vi "Stiffness Jacobian DAO.vi"(7 "refnum in":T1, 8 "error in (no error)":errorcluster, 9 "Stiffness Jacobian In":T4=[[1000000.0, 0.0, 0.0, 0.0, 0.0, 0.0], [0.0, 1000000.0, 0.0, 0.0, 0.0, 0.0], [0.0, 0.0, 1000000.0, 0.0, 0.0, 0.0], [0.0, 0.0, 0.0, 1000000.0, 0.0, 0.0], [0.0, 0.0, 0.0, 0.0, 1000000.0, 0.0], [0.0, 0.0, 0.0, 0.0, 0.0, 1000000.0]], 10 "LBCB Number":T2, 11 "Actions":T3) -> (0 "error out":errorcluster, 3 "Stiffness Jacobian Out":T4=[[1000000.0, 0.0, 0.0, 0.0, 0.0, 0.0], [0.0, 1000000.0, 0.0, 0.0, 0.0, 0.0], [0.0, 0.0, 1000000.0, 0.0, 0.0, 0.0], [0.0, 0.0, 0.0, 1000000.0, 0.0, 0.0], [0.0, 0.0, 0.0, 0.0, 1000000.0, 0.0], [0.0, 0.0, 0.0, 0.0, 0.0, 1000000.0]], 4 "refnum out":T1)   [LabVIEW 2009]
uses:
  MixedMode/Stiffness Matrix.ctl
  Metadata/Persistant DAO Actions.ctl
  Metadata/LBCB Number.ctl
  <vilib>/Utility/config.llb/Config Data RefNum.ctl
  <vilib>/Utility/config.llb/NI_LVConfig.lvlib
panel:
  in  "Keys":string[](array[string])=["dFx", "dFy", "dFz", "dMx", "dMy", "dMz"]
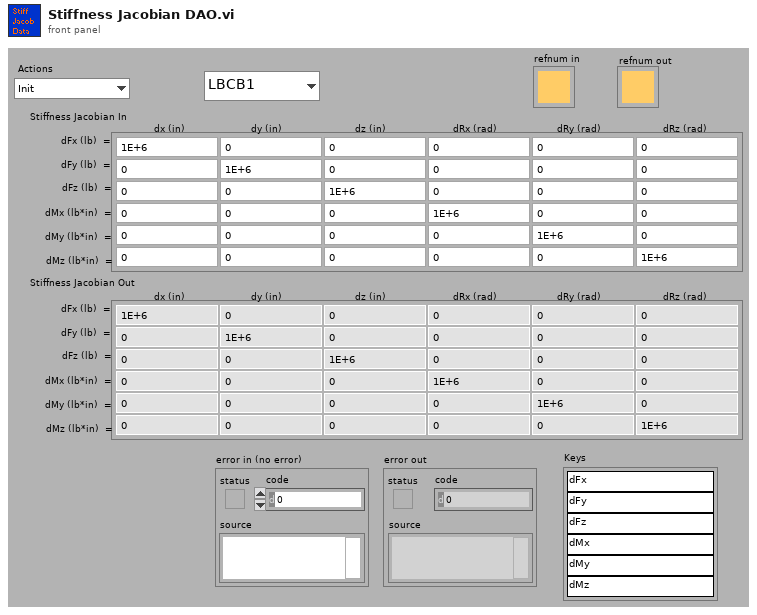
[diagram p1: front panel]
types:
  T1 = typedef "NI_LVConfig.lvlib/Config Data RefNum.ctl" = refnum<k1>
  T2 = typedef "LBCB Number.ctl" = enum16{"LBCB1", "LBCB2"}
  T3 = typedef "Persistant DAO Actions.ctl" = enum16{"Init", "Get", "Set", "Load", "Save"}
  T4 = typedef "Stiffness Matrix.ctl" = dbl[][]
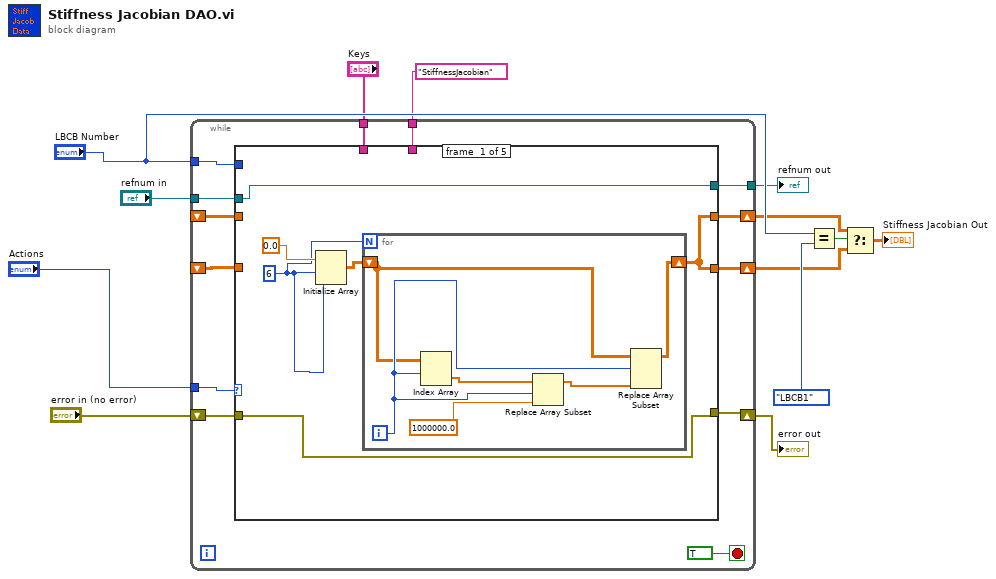
[diagram p0: block diagram]
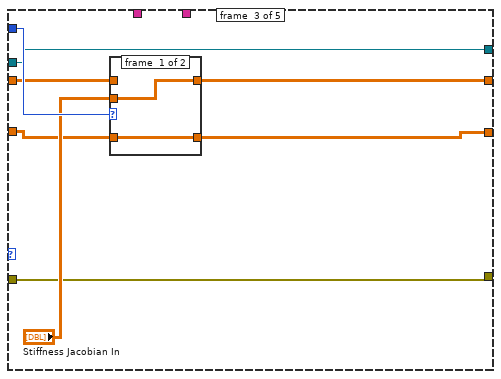
[diagram p3: hidden frame]
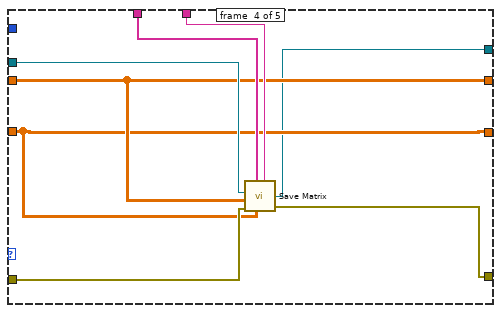
[diagram p5: hidden frame]
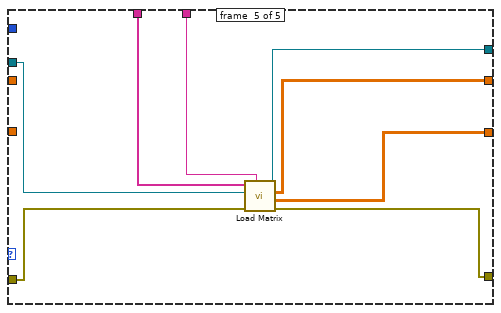
[diagram p6: hidden frame]
diagram:
  n1 = while {
    tunnel: "Actions" -> [w25]
    tunnel: "LBCB Number" -> [w24]
    shift-right: [w23] -> w8
    shift-left: _ -> [w15]
    shift-right: [w22] -> w9
    shift-left: _ -> [w14]
    tunnel: "refnum in" -> [w21]
    tunnel: [w20] -> w5
    shift-right: [w18] -> w3
    shift-left: "error in (no error)" -> [w19]
    tunnel: "StiffnessJacobian" -> [w17]
    tunnel: "Keys" -> [w16]
    stop <- TRUE stop-if-true
    n2 = case shown="\"Save\"" w25 {
      tunnel: w24 -> [_ _ w50 _ _]
      tunnel: [w29 w41 w48 w57 w66] -> w23
      tunnel: [w29 w42 w47 w58 w65] -> w22
      tunnel: w21 -> [w28 w39 w45 w62 w70]
      tunnel: [w28 w39 w45 w56 w69] -> w20
      tunnel: w19 -> [w27 w40 w43 w61 w68]
      tunnel: [w27 w40 w43 w55 w67] -> w18
      tunnel: w17 -> [_ _ _ w60 w63]
      tunnel: w16 -> [_ _ _ w59 w64]
      tunnel: w15 -> [_ w41 w44 w57 _]
      tunnel: w14 -> [_ w42 w46 w58 _]
      frame #0 {
        w31 = 6 ("dimension size")
        n3 = Initialize Array(0.0, w31, w31) -> (w30:dbl[][])
        n4 = for {
          N: w31 -> [_]
          shift-right: [w33] -> w29
          shift-left: w30 -> [w34]
          i -> [w35]
          n5 = Index Array(array=w34, index (row)=w35) -> (element=w38:dbl[])  [unwired: 1 in]
          n6 = Replace Array Subset(array=w38, new element=1000000.0 ("new element/subarray"), index=w35) -> (w36:dbl[])
          n7 = Replace Array Subset(array=w34, new element=w36, index (row)=w35) -> (w33:dbl[][])  [unwired: 1 in]
        }
      }
      frame #1 {
      }
      frame #2 {
        n8 = case shown="\"LBCB1\", Default" w50 {
          tunnel: "Stiffness Jacobian In" -> [w52 w54]
          tunnel: [w51 w54] -> w48
          tunnel: [w52 w53] -> w47
          tunnel: w46 -> [_ w53]
          tunnel: w44 -> [w51 _]
          frame #0 {
          }
          frame #1 {
          }
        }
      }
      frame #3 {
        n9 = call "Save Matrix.vi"("section"=w60, "Matrix 2"=w57, "error in (no error)"=w61, "Matrix 1"=w58, "Keys"=w59, "refnum in"=w62) -> ("error out"=w55:errorcluster, "refnum out"=w56:T1)  [unwired: 2 in, 1 out]
      }
      frame #4 {
        n10 = call "Load Matrix.vi"("section"=w63, "error in (no error) 2"=w68, "refnum in"=w70, "Keys"=w64) -> ("error in (no error)"=w67:errorcluster, "Matrix 2"=w66:dbl[][], "Matrix 1"=w65:dbl[][], "refnum out"=w69:T1)  [unwired: 4 out]
      }
    }
  }
  "error out" <- w3
  "refnum out" <- w5
  n11 = Equal?(x="LBCB Number", y=LBCB_Number."LBCB1") -> (x = y?=w12:bool)
  n12 = Select(t=w9, s=w12, f=w8) -> (s? t:f=→"Stiffness Jacobian Out":T4)
